vi "Set Palette Visible.vi"(6 "Control Ref Queue":T2, 8 "error in (no error)":errorcluster, 9 "Action ID in":u32=1, 10 "Item Tag":string, 11 "2D Plot in":refnum<class "2D Plot.lvclass">) -> (0 "error out":errorcluster, 1 "Action String":T1=1 items=["Show/Hide", "Change Attribute", "Text Edit", "Cursor Move"], 2 "State Change?":bool, 3 "2D Plot out":refnum<class "2D Plot.lvclass">, 5 "Update Legend?":bool)   [LabVIEW 2017, in "2D Plot.lvclass"]
uses:
  <vilib>/Math Plots/2D Math Plots/2D Plot/2D Plot/2D Plot.lvclass
  <vilib>/Math Plots/2D Math Plots/2D Plot/Action String/2DMathPlot Ctrl Act Queue.ctl
  <vilib>/Math Plots/2D Math Plots/2D Plot/Action String/2DMathPlot Ctrl Act Cluster.ctl
  <vilib>/Math Plots/2D Math Plots/2D Plot/Action String/2DMathPlot State Class.ctl
  <vilib>/Math Plots/2D Math Plots/2D Plot/Action String/2DMathPlot Action String.ctl
  <vilib>/Math Plots/2D Math Plots/2D Plot/2D Plot/2D Plot.lvclass/2D Plot.ctl
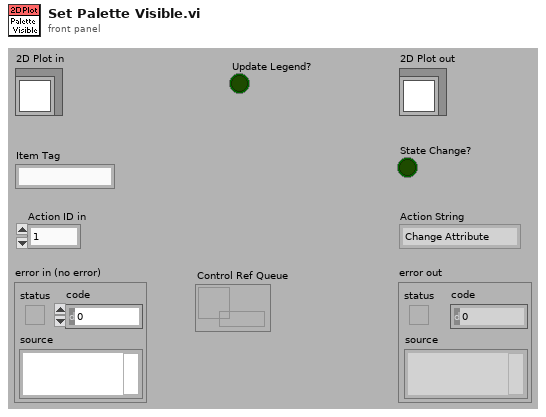
[diagram p1: front panel]
types:
  T1 = typedef "2DMathPlot Action String.ctl" = u16
  T2 = typedef "2DMathPlot Ctrl Act Queue.ctl" = refnum<queue>
  T3 = typedef "2DMathPlot Ctrl Act Cluster.ctl" = cluster{"Plot Area Ref":refnum<vi>, "Z Axis Ref":refnum<vi>, "Legend Ref":refnum<vi>, "XControl Ref":refnum<vi>, "Facade Ref":refnum<vi>, "Display State Change Class":T4}
  T4 = typedef "2DMathPlot State Class.ctl" = enum16{"Update All (Undo)", "Update General", "Update Appearance", "Update Format", "Update Scale", "Update Marker", "Update Cursor", "None"}
  T5 = typedef "2D Plot.lvclass/Scale Array.ctl" = T6[]
  T6 = typedef "2D Plot.lvclass/Scale Cluster.ctl" = cluster{"General":cluster{"Editable":bool, "Flipped":bool, "Mapping Mode":u8, "Visible":bool, "Style":u8, "Scale Fit":u8}, "Offset and Multiplier":T7, "Range":cluster{"Minimum":dbl, "Maximum":dbl, "Increment":dbl, "Minor Increment":dbl, "Start":dbl}, "Tick Color":cluster{"Major Color":u32, "Minor Color":u32}, "Gird Color":cluster{"Major Color":u32, "Minor Color":u32}, "Marker":cluster{"Visible":bool, "FG Color":u32, "BG Color":u32, "Font Name":string, "Font Size":u32, "Font Bold":bool, "Font Italic":bool, "Font Strikeout":bool, "Font Underline":bool}, "Name Label":cluster{"Visible":bool, "FG Color":u32, "BG Color":u32, "Font Name":string, "Font Size":u32, "Font Bold":bool, "Font Italic":bool, "Font Strikeout":bool, "Font Underline":bool, "Justification":enum16{"Left", "Center", "Right"}, "Text":string}}
  T7 = typedef "LVOffsetAndMultiplierTypeDef.ctl" = cluster{"Offset":dbl, "Multiplier":dbl}
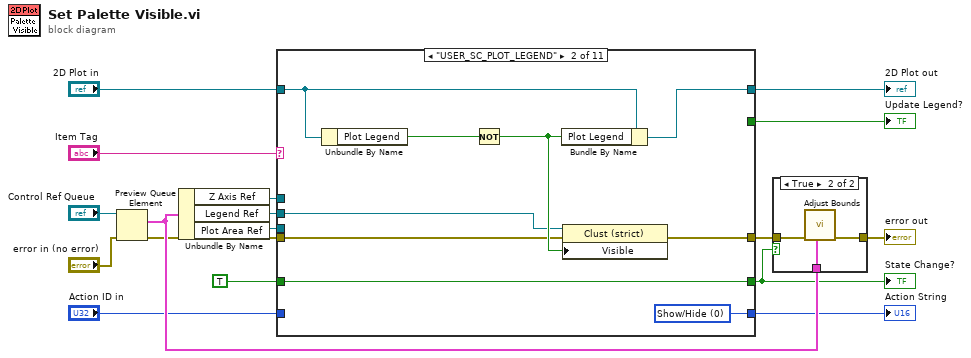
[diagram p0: block diagram]
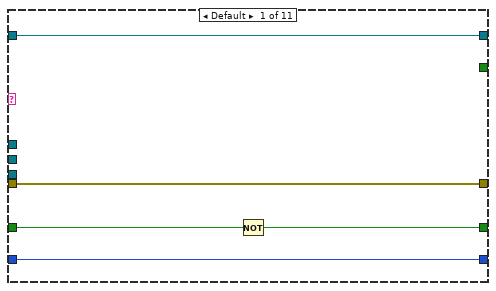
[diagram p3: hidden frame]
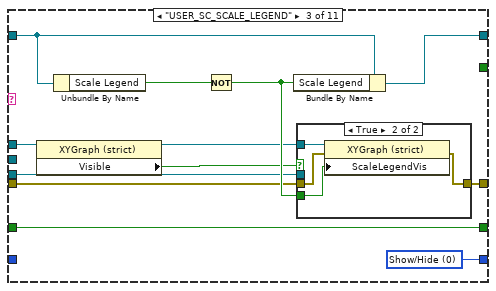
[diagram p4: hidden frame]
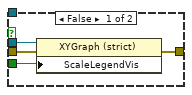
[diagram p5: hidden frame]
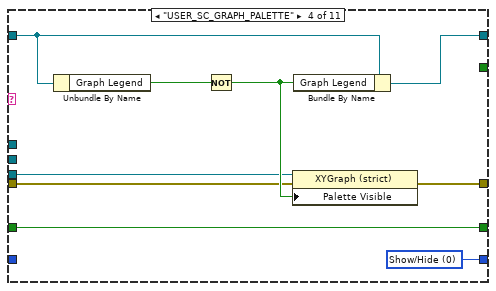
[diagram p6: hidden frame]
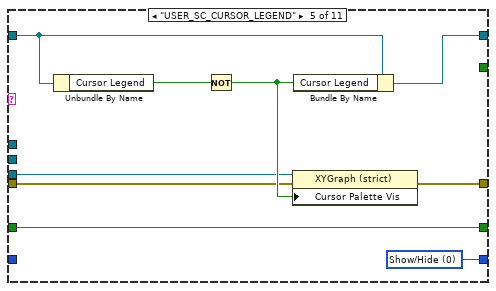
[diagram p7: hidden frame]
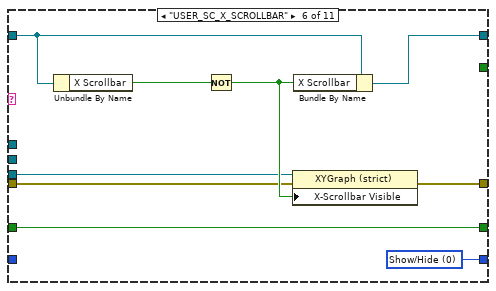
[diagram p8: hidden frame]
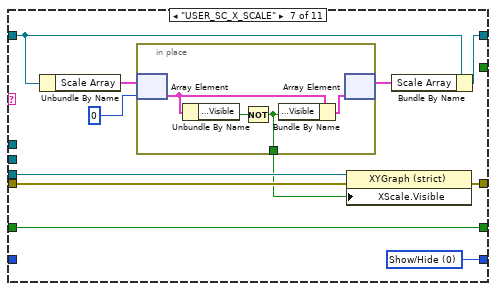
[diagram p9: hidden frame]
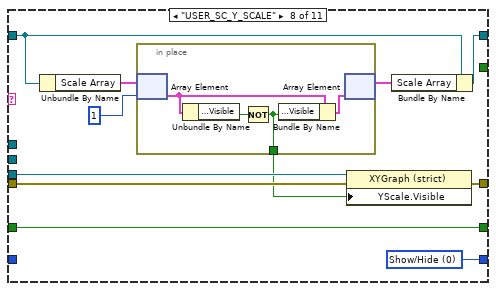
[diagram p10: hidden frame]
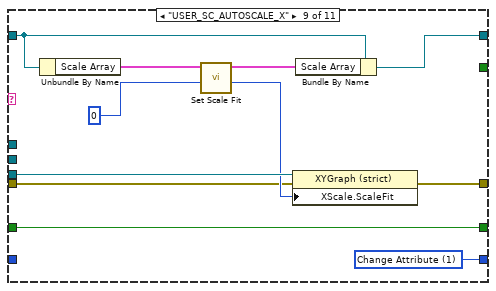
[diagram p11: hidden frame]
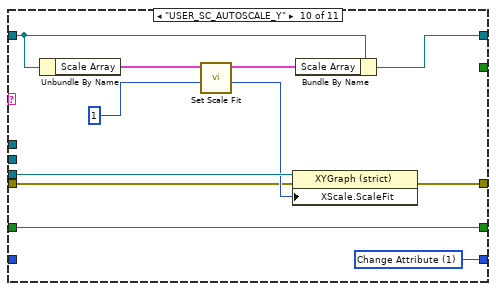
[diagram p12: hidden frame]
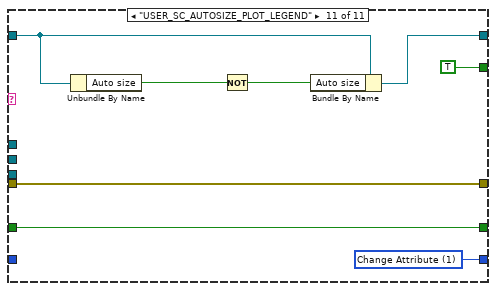
[diagram p13: hidden frame]
diagram:
  n1 = Preview Queue Element(queue="Control Ref Queue", error in (no error)="error in (no error)") -> (element=w15:T3, error out=w8:errorcluster)  [unwired: 3 out]
  n2 = Unbundle By Name(w15) -> ("Z Axis Ref"=w6:refnum<vi>, "Legend Ref"=w7:refnum<vi>, "Plot Area Ref"=w14:refnum<vi>)
  n3 = case shown="\"USER_SC_PLOT_LEGEND\"" "Item Tag" {
    tunnel: "2D Plot in" -> [w22 w29 w41 w56 w65 w76 w89 w104 w119 w130 w138]
    tunnel: [w22 w30 w38 w55 w64 w72 w88 w103 w118 w129 w135] -> w9
    tunnel: w8 -> [w21 w26 w40 w57 w66 w75 w83 w98 w111 w122 w134]
    tunnel: w14 -> [_ _ w37 w58 w67 w74 w84 w99 w114 w125 _]
    tunnel: [w21 w27 w39 w54 w63 w73 w82 w97 w112 w123 w134] -> w16
    tunnel: [w19 w23 w32 w52 w61 w70 w79 w94 w109 w120 w131] -> w3
    tunnel: w7 -> [_ w25 _ _ _ _ _ _ _ _ _]
    tunnel: w6 -> [_ _ w36 _ _ _ _ _ _ _ _]
    tunnel: [_ _ _ _ _ _ _ _ _ _ TRUE] -> w5
    tunnel: [w18 w24 w33 w53 w62 w71 w80 w95 w110 w121 w132] -> w4
    tunnel: TRUE ("State Change? in") -> [w20 w23 w32 w52 w61 w70 w79 w94 w109 w120 w131]
    tunnel: "Action ID in" -> [w18 _ _ _ _ _ _ _ _ _ _]
    frame Default {
      n4 = Not(x=w20) -> (.not. x?=w19:bool)
    }
    frame "USER_SC_PLOT_LEGEND" {
      w24 = T1 0 items=["Show/Hide", "Change Attribute", "Text Edit", "Cursor Move"] ("Global String")
      n5 = Unbundle By Name(w29) -> ("Plot Legend"=w31:bool)
      n6 = Not(x=w31) -> (.not. x?=w28:bool)
      n7 = Bundle By Name(cluster=w29, "Plot Legend"=w28) -> (w30:refnum<class "2D Plot.lvclass">)
      n8 = property class="Clust (strict)"(reference=w25, error in=w26, "Visible"=w28) -> (error out=w27:errorcluster)  [unwired: 1 out]
    }
    frame "USER_SC_SCALE_LEGEND" {
      w33 = T1 0 items=["Show/Hide", "Change Attribute", "Text Edit", "Cursor Move"] ("Global String")
      n9 = property class="XYGraph (strict)"(reference=w36) -> (reference out=w34:refnum<vi>, "Visible"=w35:bool)  [unwired: 1 in, 1 out]
      n10 = Unbundle By Name(w41) -> ("Scale Legend"=w43:bool)
      n11 = Not(x=w43) -> (.not. x?=w42:bool)
      n12 = Bundle By Name(cluster=w41, "Scale Legend"=w42) -> (w38:refnum<class "2D Plot.lvclass">)
      n13 = case shown="True" w35 {
        tunnel: w42 -> [w47 w48]
        tunnel: w40 -> [w46 w50]
        tunnel: [w45 w49] -> w39
        tunnel: w37 -> [w44 _]
        tunnel: w34 -> [_ w51]
        frame False {
          n14 = property class="XYGraph (strict)"(reference=w44, error in=w46, "ScaleLegendVis"=w47) -> (error out=w45:errorcluster)  [unwired: 1 out]
        }
        frame True {
          n15 = property class="XYGraph (strict)"(reference=w51, error in=w50, "ScaleLegendVis"=w48) -> (error out=w49:errorcluster)  [unwired: 1 out]
        }
      }
    }
    frame "USER_SC_GRAPH_PALETTE" {
      w53 = T1 0 items=["Show/Hide", "Change Attribute", "Text Edit", "Cursor Move"] ("Global String")
      n16 = Unbundle By Name(w56) -> ("Graph Legend"=w60:bool)
      n17 = Not(x=w60) -> (.not. x?=w59:bool)
      n18 = property class="XYGraph (strict)"(reference=w58, error in=w57, "Palette Visible"=w59) -> (error out=w54:errorcluster)  [unwired: 1 out]
      n19 = Bundle By Name(cluster=w56, "Graph Legend"=w59) -> (w55:refnum<class "2D Plot.lvclass">)
    }
    frame "USER_SC_CURSOR_LEGEND" {
      w62 = T1 0 items=["Show/Hide", "Change Attribute", "Text Edit", "Cursor Move"] ("Global String")
      n20 = Unbundle By Name(w65) -> ("Cursor Legend"=w69:bool)
      n21 = Not(x=w69) -> (.not. x?=w68:bool)
      n22 = property class="XYGraph (strict)"(reference=w67, error in=w66, "Cursor Palette Vis"=w68) -> (error out=w63:errorcluster)  [unwired: 1 out]
      n23 = Bundle By Name(cluster=w65, "Cursor Legend"=w68) -> (w64:refnum<class "2D Plot.lvclass">)
    }
    frame "USER_SC_X_SCROLLBAR" {
      w71 = T1 0 items=["Show/Hide", "Change Attribute", "Text Edit", "Cursor Move"] ("Global String")
      n24 = Unbundle By Name(w76) -> ("X Scrollbar"=w78:bool)
      n25 = Not(x=w78) -> (.not. x?=w77:bool)
      n26 = property class="XYGraph (strict)"(reference=w74, error in=w75, "X-Scrollbar Visible"=w77) -> (error out=w73:errorcluster)  [unwired: 1 out]
      n27 = Bundle By Name(cluster=w76, "X Scrollbar"=w77) -> (w72:refnum<class "2D Plot.lvclass">)
    }
    frame "USER_SC_X_SCALE" {
      w80 = T1 0 items=["Show/Hide", "Change Attribute", "Text Edit", "Cursor Move"] ("Global String")
      n28 = Unbundle By Name(w89) -> ("Scale Array"=w87:T5)
      n29 = in-place {
        in-place-border: [w90] -> w81
        n30 = in-place-array #1(w87, 0) -> (w93:T6)
        n31 = Unbundle By Name(w93) -> ("General.Visible"=w91:bool)
        n32 = Not(x=w91) -> (.not. x?=w90:bool)
        n33 = Bundle By Name(cluster=w93, "General.Visible"=w90) -> (w92:T6)
        n34 = in-place-array #1(w92) -> (w86:T5)  [unwired: 1 out]
      }
      n35 = property class="XYGraph (strict)"(reference=w84, error in=w83, "XScale.Visible"=w81) -> (error out=w82:errorcluster)  [unwired: 1 out]
      n36 = Bundle By Name(cluster=w89, "Scale Array"=w86) -> (w88:refnum<class "2D Plot.lvclass">)
    }
    frame "USER_SC_Y_SCALE" {
      w95 = T1 0 items=["Show/Hide", "Change Attribute", "Text Edit", "Cursor Move"] ("Global String")
      n37 = Unbundle By Name(w104) -> ("Scale Array"=w102:T5)
      n38 = in-place {
        in-place-border: [w105] -> w96
        n39 = in-place-array #2(w102, 1) -> (w108:T6)
        n40 = Unbundle By Name(w108) -> ("General.Visible"=w106:bool)
        n41 = Not(x=w106) -> (.not. x?=w105:bool)
        n42 = Bundle By Name(cluster=w108, "General.Visible"=w105) -> (w107:T6)
        n43 = in-place-array #2(w107) -> (w101:T5)  [unwired: 1 out]
      }
      n44 = property class="XYGraph (strict)"(reference=w99, error in=w98, "YScale.Visible"=w96) -> (error out=w97:errorcluster)  [unwired: 1 out]
      n45 = Bundle By Name(cluster=w104, "Scale Array"=w101) -> (w103:refnum<class "2D Plot.lvclass">)
    }
    frame "USER_SC_AUTOSCALE_X" {
      w110 = T1 1 items=["Show/Hide", "Change Attribute", "Text Edit", "Cursor Move"] ("Global String")
      n46 = Unbundle By Name(w119) -> ("Scale Array"=w117:T5)
      n47 = call <vilib>:"Set Scale Fit.vi"("Axis Index"=0, "Scale Array In"=w117) -> ("Scale Fit"=w113:u8, "Scale Array Out"=w116:T5)  [unwired: 8 out]
      n48 = property class="XYGraph (strict)"(reference=w114, error in=w111, "XScale.ScaleFit"=w113) -> (error out=w112:errorcluster)  [unwired: 1 out]
      n49 = Bundle By Name(cluster=w119, "Scale Array"=w116) -> (w118:refnum<class "2D Plot.lvclass">)
    }
    frame "USER_SC_AUTOSCALE_Y" {
      w121 = T1 1 items=["Show/Hide", "Change Attribute", "Text Edit", "Cursor Move"] ("Global String")
      n50 = Unbundle By Name(w130) -> ("Scale Array"=w128:T5)
      n51 = call <vilib>:"Set Scale Fit.vi"("Axis Index"=1, "Scale Array In"=w128) -> ("Scale Fit"=w124:u8, "Scale Array Out"=w127:T5)  [unwired: 8 out]
      n52 = property class="XYGraph (strict)"(reference=w125, error in=w122, "XScale.ScaleFit"=w124) -> (error out=w123:errorcluster)  [unwired: 1 out]
      n53 = Bundle By Name(cluster=w130, "Scale Array"=w127) -> (w129:refnum<class "2D Plot.lvclass">)
    }
    frame "USER_SC_AUTOSIZE_PLOT_LEGEND" {
      w132 = T1 1 items=["Show/Hide", "Change Attribute", "Text Edit", "Cursor Move"] ("Global String")
      n54 = Unbundle By Name(w138) -> ("Auto size"=w137:bool)
      n55 = Not(x=w137) -> (.not. x?=w136:bool)
      n56 = Bundle By Name(cluster=w138, "Auto size"=w136) -> (w135:refnum<class "2D Plot.lvclass">)
    }
  }
  "2D Plot out" <- w9
  "State Change?" <- w3
  "Update Legend?" <- w5
  "Action String" <- w4
  n57 = case shown="True" w3 {
    tunnel: w16 -> [w139 w142]
    tunnel: w15 -> [_ w141]
    tunnel: [w139 w140] -> w12
    frame False {
    }
    frame True {
      n58 = call <vilib>:"Adjust Bounds.vi"("Control Ref Cluster"=w141, "error in (no error)"=w142) -> ("error out"=w140:errorcluster)  [unwired: 9 out]
    }
  }
  "error out" <- w12
